vi "UDP_buffer_Example.vi"() -> ()   [LabVIEW 2010]
doc: "Shows a use of the UDP_Set_Receive_Buffer_Size.vi."
panel:
  out "Actual Rx Buffer Size (bytes)":u32
  in  "Bytes to Read":u32=1024
  in  "Port":u16=1234
  out "data out":string
  in  "Set Rx Buffer Size (bytes)":u32=8192
  # "InstructionsL\n     1) Set the port, number of bytes to read, and \n             receive buffer size.\n     2) Run the VI.\n     2) Send UDP packets to the port specified."
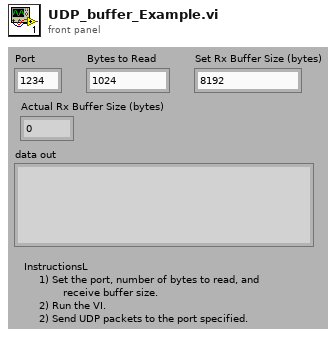
[diagram p1: front panel]
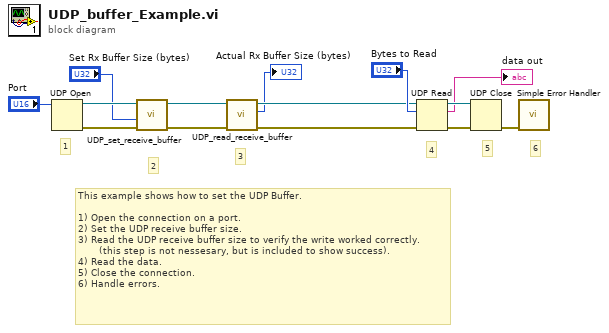
[diagram p0: block diagram]
diagram:
  # "6"
  # "3"
  # "This example shows how to set the UDP Buffer.\n\n1) Open the connection on a port.\n2) Set the UDP receive buffer size.\n3) Read the UDP receive buffer size to verify the write worked correctly.\n       (this step is not nessesary, but is included to show success).\n4) Read the data.\n5) Close the connection.\n6) Handle errors."
  # "5"
  # "4"
  # "2"
  # "1"
  n1 = UDP Open(11:"Port") -> (port=w14:refnum<k16>, 0:w13:errorcluster)  [unwired: 4 in, 1 out]
  n2 = call "UDP_set_receive_buffer.vi"("error in (no error)"=w13, "Receive Buffer Size"="Set Rx Buffer Size (bytes)", "connection ID"=w14) -> ("error out"=w4:errorcluster, "connection ID out"=w5:refnum<k16>)  [unwired: 6 in]
  n3 = call "UDP_read_receive_buffer.vi"("error in (no error)"=w4, "connection ID"=w5) -> ("error out"=w3:errorcluster, "Receive Buffer Size"=→"Actual Rx Buffer Size (bytes)":u32, "connection ID out"=w2:refnum<k16>)  [unwired: 5 in]
  n4 = UDP Read(connection ID=w2, max size (548)="Bytes to Read", 8:w3) -> (data out=→"data out":string, error out=w11:errorcluster, 3:w10:refnum<k16>)  [unwired: 1 in, 2 out]
  n5 = UDP Close(connection ID=w10, 8:w11) -> (error out=w9:errorcluster)  [unwired: 1 out]
  n6 = call <vilib>:"Simple Error Handler.vi"("error in (no error)"=w9) -> ()  [unwired: 4 in, 5 out]
